vi "Get_Width.vi"(8 "error in (no error)":errorcluster caption="错误输入（无错误）", 11 "Size输入":refnum<class "Size.lvclass">) -> (0 "error out":errorcluster caption="错误输出", 2 "Width":dbl, 3 "Size输出":refnum<class "Size.lvclass">)   [LabVIEW 2011, in "Size.lvclass"]
uses:
  Size.lvclass
  Size.lvclass/Size.ctl
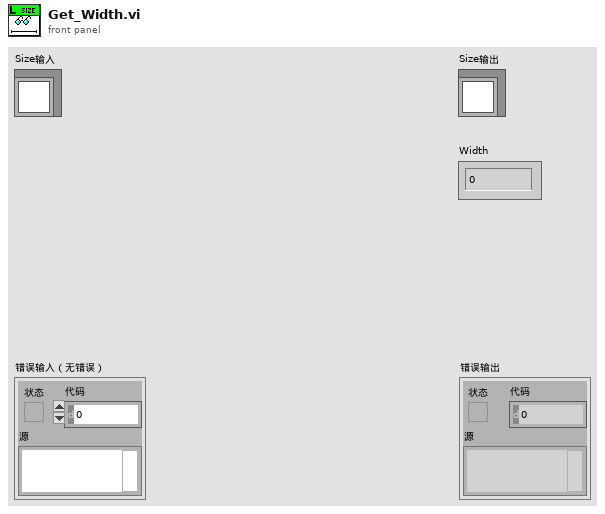
[diagram p1: front panel]
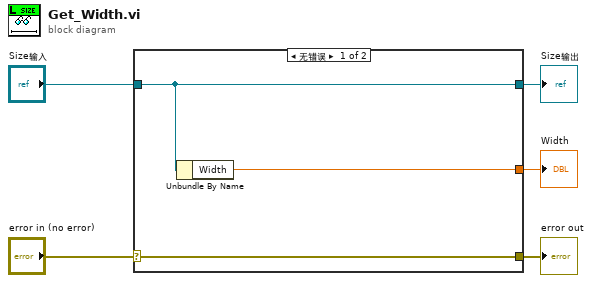
[diagram p0: block diagram]
diagram:
  n1 = case shown="无错误" "error in (no error)" {
    selector: "error in (no error)" -> [w8 w9]
    tunnel: [w8 w9] -> w4
    tunnel: [w7 w10] -> w2
    tunnel: "Size输入" -> [w7 w10]
    tunnel: [w6 _] -> w1
    frame No Error {
      n2 = Unbundle By Name(w7) -> ("Width"=w6:dbl)
    }
    frame Error {
    }
  }
  "error out" <- w4
  "Size输出" <- w2
  "Width" <- w1
